vi "Error Query.vi"(6 "Ignored Warnings":string[](array[string]), 7 "Warnings as Errors":string[](array[string]), 8 "error in (no error)":errorcluster, 9 "Device and Axis":string, 10 "Previous Response Bundle Array":T1(array[cluster]), 11 "VISA resource name":refnum<visa-resource-name>) -> (0 "error out":errorcluster, 1 "Error Message":string, 2 "Error Code":i32, 3 "VISA resource name out":refnum<visa-resource-name>)   [LabVIEW 2018, in "Zaber A Series.lvlib"]
doc: "Checks a collection of responses for warning flags and reports all warnings from responding devices that have warning conditions.\n\nOptional inputs allow for ignoring some warnings or treating some warnings as error conditions. Both of these inputs are arrays of strings, each of which should be a two-letter warning code as seen in the Zaber ASCII Protocol Manual at http://www.zaber.com/wiki/Manuals/ASCII_Protocol_Manual#Warning_Flags. \n\nYou can globally ignore warnings or treat warnings as errors without having to wire up the relevant inputs everywhere by entering new defaults for the inputs - see the note on this VI's front panel.\n\nThis VI requires that the Initialize VI has been called with the same serial port."
uses:
  Zaber A Series.lvlib
  Private/All Commands.ctl
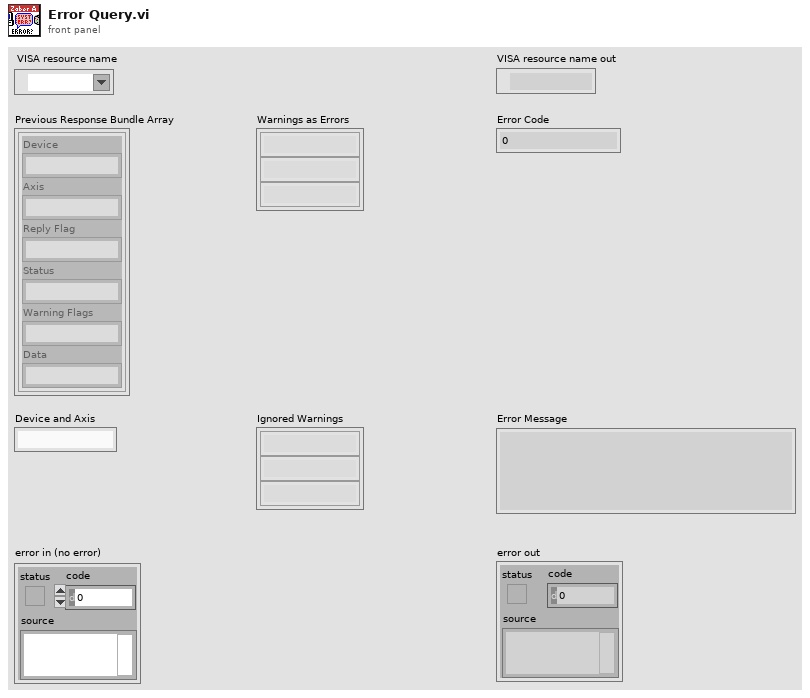
[diagram p1: front panel]
types:
  T1 = cluster{"Device":string, "Axis":string, "Reply Flag":string, "Status":string, "Warning Flags":string, "Data":string}[]
  T2 = typedef "Zaber A Series.lvlib/All Commands.ctl" = string
  T3 = cluster{"Device":string, "Axis":string, "Reply Flag":string, "Status":string, "Warning Flags":string, "Data":string}
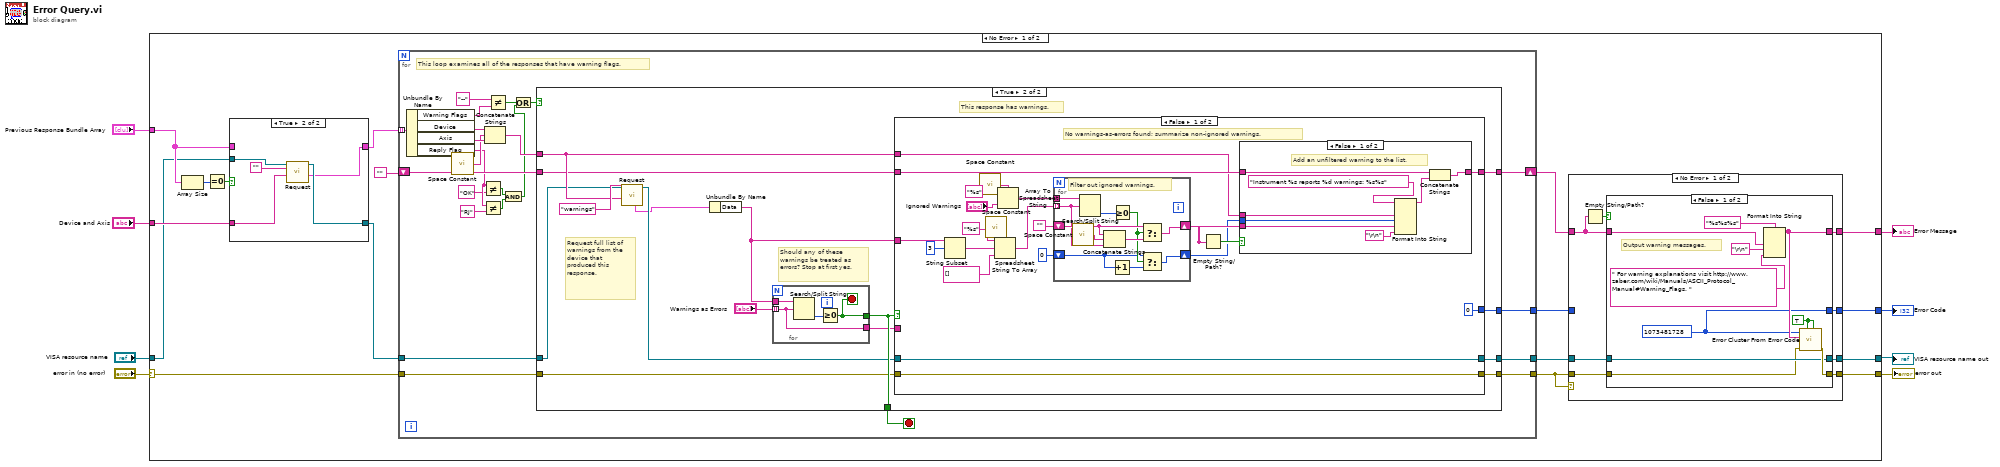
[diagram p0: block diagram]
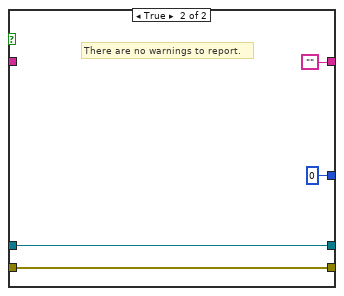
[diagram p3: hidden frame]
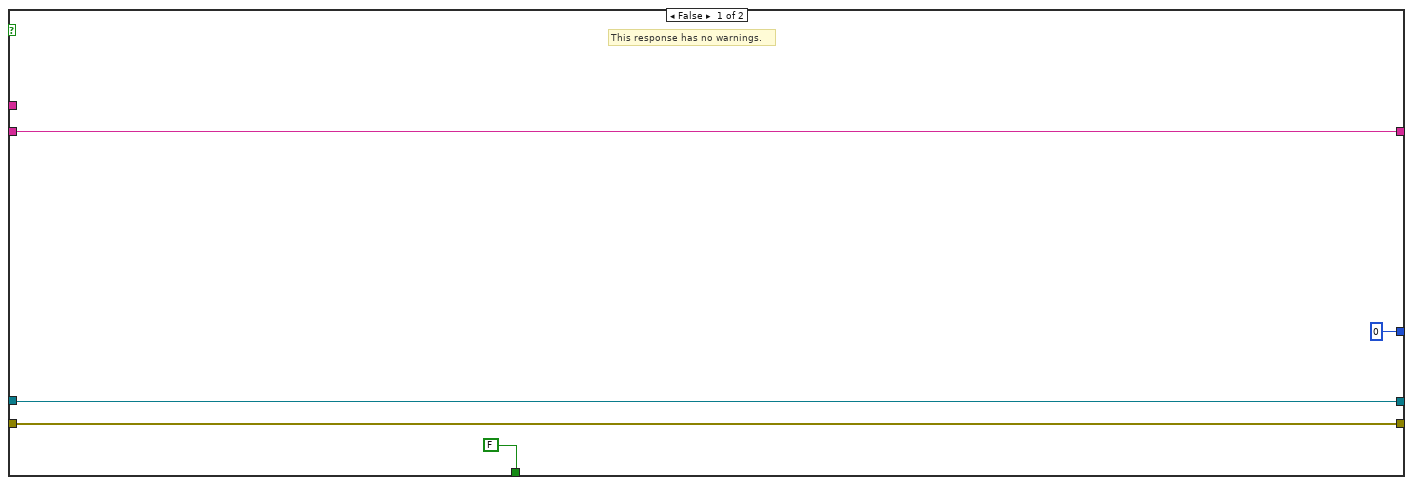
[diagram p5: hidden frame]
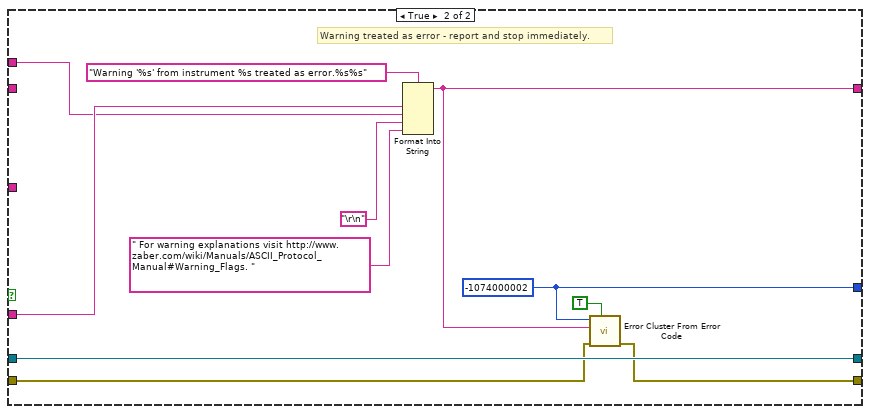
[diagram p7: hidden frame]
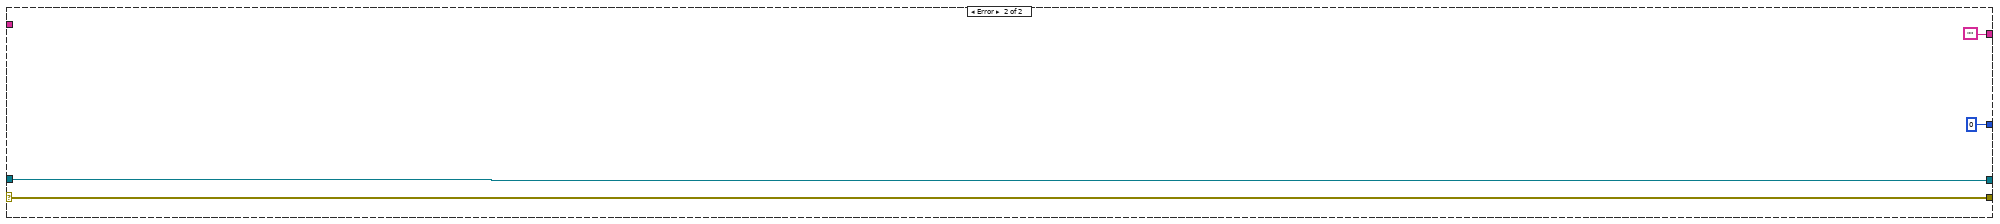
[diagram p8: hidden frame]
diagram:
  n1 = case shown="No Error" "error in (no error)" {
    selector: "error in (no error)" -> [w21 w161]
    tunnel: [w23 w162] -> w8
    tunnel: "VISA resource name" -> [w10 w162]
    tunnel: [w24 w161] -> w4
    tunnel: [w22 ""] -> w2
    tunnel: [w25 0 ("Code")] -> w5
    tunnel: "Device and Axis" -> [w11 _]
    tunnel: "Previous Response Bundle Array" -> [w13 _]
    frame No Error {
      n2 = Array Size(array=w13) -> (size(s)=w20:i32)
      n3 = Equal To 0?(x=w20) -> (x = 0?=w14:bool)
      n4 = case shown="True" w14 {
        tunnel: w13 -> [w27 _]
        tunnel: [w27 w28] -> w12
        tunnel: w11 -> [_ w32]
        tunnel: w10 -> [w26 w30]
        tunnel: [w26 w29] -> w9
        frame False {
        }
        frame True {
          n5 = call "Request.vi"("Device and Axis"=w32, "Command String"="", "VISA resource name"=w30) -> ("Response Bundle Array"=w28:T1, "VISA resource name out"=w29:refnum<visa-resource-name>)  [unwired: 3 in, 4 out]
        }
      }
      n6 = for {
        tunnel: w21 -> [w77]
        tunnel: [w81] -> w16
        tunnel: w12 -> [w76] mode=indexing
        tunnel: w9 -> [w79]
        tunnel: [w78] -> w17
        shift-right: [w67] -> w19
        shift-left: "" -> [w68]
        tunnel: [w80] -> w15
        stop <- w69 stop-if-true
        # "This loop examines all of the responses that have warning flags."
        n7 = Unbundle By Name(w76) -> ("Warning Flags"=w74:string, "Device"=w73:string, "Axis"=w72:string, "Reply Flag"=w66:string)
        n8 = call <vilib>:"Space Constant.vi"() -> ("String"=w71:string)
        n9 = Not Equal?(x=w66, y="OK") -> (x != y?=w63:bool)
        n10 = Not Equal?(x=w66, y="RJ") -> (x != y?=w62:bool)
        n11 = Concatenate Strings(w73, w71, w72) -> (w70:string)
        n12 = Not Equal?(x="--", y=w74) -> (x != y?=w60:bool)
        n13 = And(x=w63, y=w62) -> (x .and. y?=w59:bool)
        n14 = Or(x=w60, y=w59) -> (x .or. y?=w61:bool)
        n15 = case shown="True" w61 {
          tunnel: [w86 w101] -> w81
          tunnel: [0 ("error code (0)") w96] -> w80
          tunnel: w79 -> [w85 w88]
          tunnel: [w85 w97] -> w78
          tunnel: w77 -> [w86 w90]
          tunnel: w70 -> [_ w94]
          tunnel: [FALSE w99] -> w69
          tunnel: w68 -> [w83 w92]
          tunnel: [w83 w89] -> w67
          frame False {
            # "This response has no warnings."
          }
          frame True {
            # "This response has warnings."
            # "Should any of these warnings be treated as errors? Stop at first yes."
            # "Request full list of warnings from the device that produced this response."
            n16 = call "Request.vi"("Device and Axis"=w94, "Command String"=T2 "warnings" ("Warning Command"), "VISA resource name"=w88) -> ("VISA resource name out"=w98:refnum<visa-resource-name>, "First Response Bundle"=w87:T3)  [unwired: 3 in, 4 out]
            n17 = Unbundle By Name(w87) -> ("Data"=w93:string)
            n18 = for {
              tunnel: "Warnings as Errors" -> [w102] mode=indexing
              tunnel: w93 -> [w105]
              tunnel: [w103] -> w99
              tunnel: [w102] -> w95
              stop <- w103 stop-if-true
              n19 = Search/Split String(string=w105, search string/char (-)=w102) -> (offset of match=w104:i32)  [unwired: 1 in, 2 out]
              n20 = Greater Or Equal To 0?(x=w104) -> (x >= 0?=w103:bool)
            }
            n21 = case shown="False" w99 {
              tunnel: [w125 w157] -> w101
              tunnel: [0 ("error code (0)") w156] -> w96
              tunnel: w90 -> [w125 w148]
              tunnel: w98 -> [w126 w158]
              tunnel: [w126 w158] -> w97
              tunnel: w95 -> [_ w153]
              tunnel: w94 -> [w110 w152]
              tunnel: w93 -> [w124 _]
              tunnel: w92 -> [w111 _]
              tunnel: [w107 w149] -> w89
              frame False {
                # "No warnings-as-errors found; summarize non-ignored warnings."
                n22 = String Subset(string=w124, offset (0)=3) -> (substring=w120:string)  [unwired: 1 in]
                n23 = call <vilib>:"Space Constant.vi"() -> ("String"=w123:string)
                n24 = call <vilib>:"Space Constant.vi"() -> ("String"=w118:string)
                n25 = Spreadsheet String To Array(delimiter (Tab)=w118, format string="%s", spreadsheet string=w120, array type (2D Dbl)=string[] []) -> (array=w116:string[])
                n26 = Array To Spreadsheet String(delimiter (Tab)=w123, array="Ignored Warnings", 3:"%s" ("format string")) -> (spreadsheet string=w115:string)
                n27 = for {
                  tunnel: w116 -> [w141] mode=indexing
                  tunnel: w115 -> [w147]
                  shift-right: [w144] -> w112
                  shift-left: "" -> [w143]
                  shift-right: [w139] -> w108
                  shift-left: 0 -> [w137]
                  # "Filter out ignored warnings."
                  n28 = call <vilib>:"Space Constant.vi"() -> ("String"=w142:string)
                  n29 = Search/Split String(string=w147, search string/char (-)=w141) -> (offset of match=w146:i32)  [unwired: 1 in, 2 out]
                  n30 = Concatenate Strings(w143, w142, w141) -> (w145:string)
                  n31 = Increment(x=w137) -> (x+1=w138:i32)
                  n32 = Greater Or Equal To 0?(x=w146) -> (x >= 0?=w140:bool)
                  n33 = Select(t=w137, s=w140, f=w138) -> (s? t:f=w139:i32)
                  n34 = Select(t=w143, s=w140, f=w145) -> (s? t:f=w144:string)
                }
                n35 = Empty String/Path?(string/path=w112) -> (empty?=w113:bool)
                n36 = case shown="False" w113 {
                  tunnel: w112 -> [w131 _]
                  tunnel: [w129 w136] -> w107
                  tunnel: w111 -> [w134 w136]
                  tunnel: w110 -> [w133 _]
                  tunnel: w108 -> [w130 _]
                  frame False {
                    # "Add an unfiltered warning to the list."
                    n37 = Format Into String(format string="Instrument %s reports %d warnings: %s%s", w133, w130, w131, "\r\n") -> (resulting string=w135:string)  [unwired: 2 in, 1 out]
                    n38 = Concatenate Strings(w134, w135) -> (w129:string)
                  }
                  frame True {
                    # "No unfiltered warnings from this device."
                  }
                }
              }
              frame True {
                w156 = -1074000002 ("error code (0)")
                # "Warning treated as error - report and stop immediately."
                n39 = Format Into String(format string="Warning '%s' from instrument %s treated as error.%s%s", w153, w152, "\r\n", " For warning explanations visit http://www.zaber.com/wiki/Manuals/ASCII_Protocol_Manual#Warning_Flags. " ("string")) -> (resulting string=w149:string)  [unwired: 2 in, 1 out]
                n40 = call <vilib>:"Error Cluster From Error Code.vi"("show call chain? (False)"=TRUE, "error in (no error)"=w148, "error message (\"\")"=w149, "error code (0)"=w156) -> ("error out"=w157:errorcluster)  [unwired: 5 in]
              }
            }
          }
        }
      }
      n41 = case shown="No Error" w16 {
        tunnel: w17 -> [w35 w58]
        tunnel: [w34 w58] -> w23
        tunnel: w16 -> [w36 w57]
        tunnel: [w39 w57] -> w24
        tunnel: w15 -> [_ w55]
        tunnel: w19 -> [w38 w56]
        tunnel: [w40 w56] -> w22
        tunnel: [w33 w55] -> w25
        frame No Error {
          n42 = Empty String/Path?(string/path=w38) -> (empty?=w37:bool)
          n43 = case shown="False" w37 {
            tunnel: [w46 ""] -> w40
            tunnel: [w45 w54] -> w39
            tunnel: w38 -> [w44 _]
            tunnel: w36 -> [w42 w54]
            tunnel: w35 -> [w43 w53]
            tunnel: [w43 w53] -> w34
            tunnel: [w41 0 ("Code")] -> w33
            frame False {
              w41 = 1073481728 ("Code")
              w50 = TRUE ("show call chain? (False)")
              # "Output warning messages."
              n44 = Format Into String(format string="%s%s%s", w44, "\r\n", " For warning explanations visit http://www.zaber.com/wiki/Manuals/ASCII_Protocol_Manual#Warning_Flags. " ("string")) -> (resulting string=w46:string)  [unwired: 2 in, 1 out]
              n45 = call <vilib>:"Error Cluster From Error Code.vi"("is warning? (False)"=w50, "show call chain? (False)"=w50, "error in (no error)"=w42, "error message (\"\")"=w46, "error code (0)"=w41) -> ("error out"=w45:errorcluster)  [unwired: 4 in]
            }
            frame True {
              # "There are no warnings to report."
            }
          }
        }
        frame Error {
          # "In this case the error message and code outputs\nare only set if this VI generated the error."
          # "An error has already been generated; do not report warnings."
        }
      }
    }
    frame Error {
    }
  }
  "VISA resource name out" <- w8
  "Error Message" <- w2
  "Error Code" <- w5
  "error out" <- w4
